vi "Get Identifier.vi"(11 "Action Point in":refnum<class "Action Point.lvclass">) -> (2 "Identifier":string, 3 "Action Point out":refnum<class "Action Point.lvclass">)   [LabVIEW 2024, in "Action Point.lvclass"]
uses:
  Action Point.lvclass
  Action Point.lvclass/Action Point.ctl
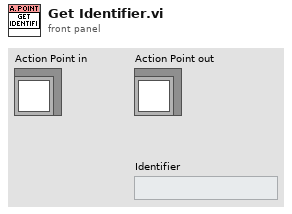
[diagram p1: front panel]
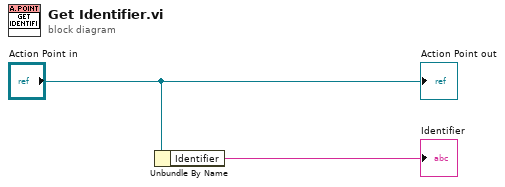
[diagram p0: block diagram]
diagram:
  n1 = Unbundle By Name("Action Point in") -> ("Identifier"=→"Identifier":string)
  "Action Point out" <- "Action Point in"
